vi "create_tree.vi"() -> ()   [LabVIEW 2021]
panel:
  out "All Tags":string[](array[string])
  out "right":string="aaa"
  out "left":string="aaa"
  out "value":i32
  in  "Tree":string(tree)
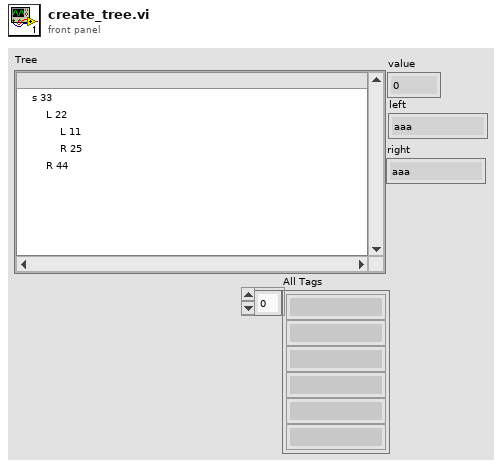
[diagram p1: front panel]
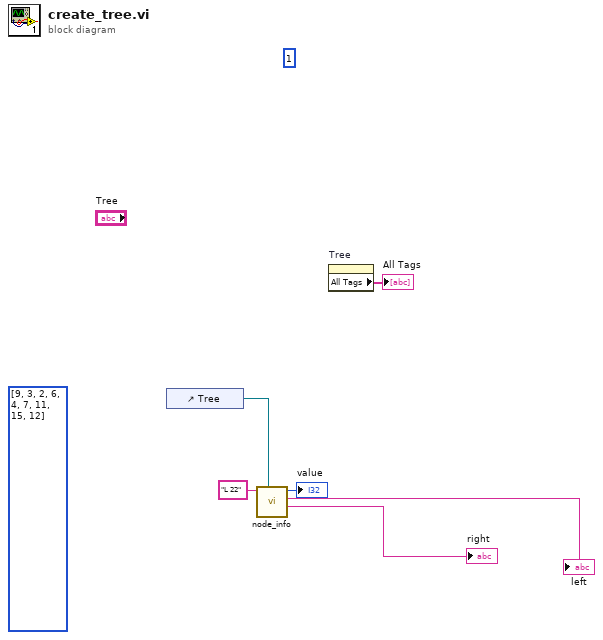
[diagram p0: block diagram]
diagram:
  (unwired) 1
  (unwired) i32[] [9, 3, 2, 6, 4, 7, 11, 15, 12]
  n1 = control-ref of="Tree"() -> (w6:refnum<vi>)
  n2 = call "node_info.vi"("reference"=w6, "node"="L 22") -> ("right"=→"right":string, "left"=→"left":string, "value"=→"value":i32)  [unwired: 6 in, 1 out]
  n3 = property on="Tree" class="Tree (strict)"() -> ("All Tags"=→"All Tags":string[])  [unwired: 2 in, 2 out]
